vi "PAM Reset Array.vi"() -> ()   [LabVIEW 2020, in "PAM Library.lvlib"]
uses:
  PAM Library.lvlib
panel:
  in  "PAM Reset Array":bool
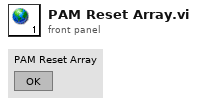
[diagram p1: front panel]
diagram:
